vi "BRig_dataLC_Loop2_c.vi"() -> (2 "output_Loop2_c":i32)   [LabVIEW 2014]
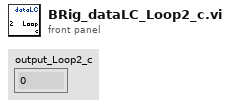
[diagram p1: front panel]
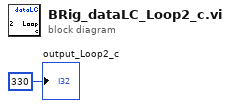
[diagram p0: block diagram]
diagram:
  "output_Loop2_c" <- 330 ("output_iBlock")
